vi "Math_Multiply_FXP.vi"(1 "y":fxp<+/-,32,16> format="%#_32g", 2 "x":fxp<+/-,32,16> format="%#_32g") -> (0 "x*y":fxp<+/-,32,16>)   [LabVIEW 2020]
uses:
  <vilib>/rvi/FXPMathLib/FxpMul/XNode/nifxpmath_Multiplier.xnode
  <vilib>/rvi/FXPMathLib/sim/FxpSim.dll
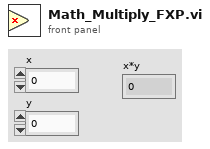
[diagram p1: front panel]
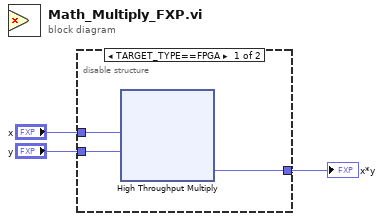
[diagram p0: block diagram]
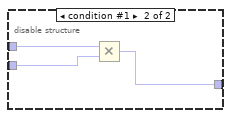
[diagram p2: hidden frame]
diagram:
  n1 = disable-structure shown="TARGET_TYPE==FPGA" {
    disable-tunnel: "x" -> [w6 w9]
    disable-tunnel: "y" -> [w5 w8]
    disable-tunnel: [w4 w7] -> w1
    frame condition #0 (active) {
      n2 = xnode ("High Throughput Multiply")("x"=w6, "y"=w5) -> ("x*y"=w4:fxp<+/-,32,16>)
    }
    frame condition #1 {
      n3 = Multiply(x=w9, y=w8) -> (x*y=w7:fxp<+/-,32,16>)
    }
  }
  "x*y" <- w1
